vi "CMI ADS127L21 - Get Error.vi"(8 "error in (no error)":errorcluster, 10 "Read All? (true)":bool=TRUE, 11 "VISA in":refnum<visa-resource-name>) -> (0 "error out":errorcluster, 3 "VISA out":refnum<visa-resource-name>)   [LabVIEW 2020]
doc: "Open digitizer."
uses:
  <vilib>/Instr/_visa.llb/VISA Flush IO Buffer Mask.ctl
  <vilib>/Utility/error.llb/Error Cluster From Error Code.vi
  <vilib>/ErrorRing/Error Ring.xnode
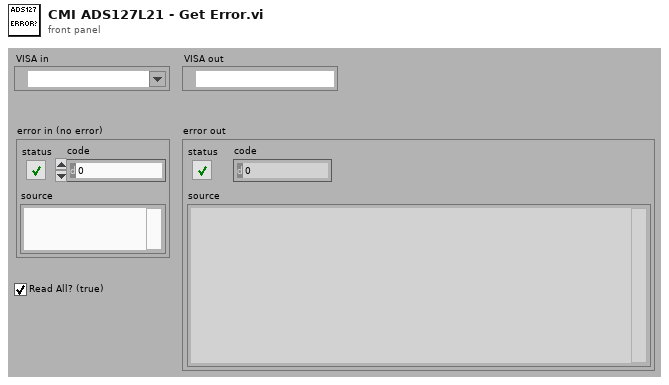
[diagram p1: front panel]
types:
  T1 = typedef "VISA Flush IO Buffer Mask.ctl" = u16
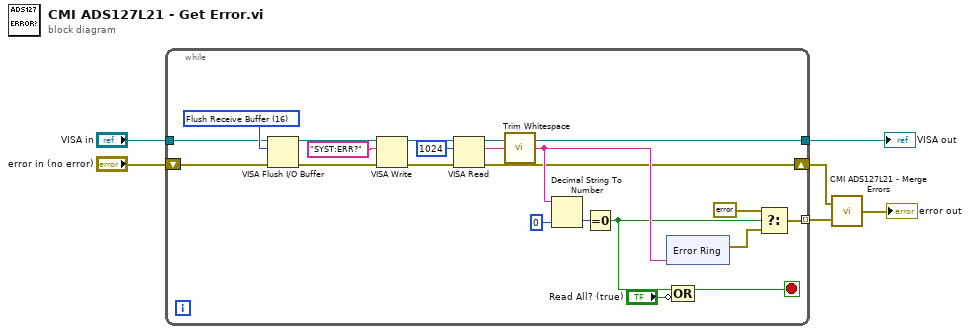
[diagram p0: block diagram]
diagram:
  n1 = while {
    tunnel: "VISA in" -> [w18]
    tunnel: [w11] -> w4 mode=indexing
    shift-right: [w12] -> w2
    shift-left: "error in (no error)" -> [w19]
    tunnel: [w10] -> w1
    stop <- w8 stop-if-true
    w27 = T1 16 items=["Flush Receive Buffer"=16, "Write Transmit Buffer to Device"=32, "Flush Receive Buffer (No I/O)"=64, "Flush Transmit Buffer"=128] ("Mask")
    n2 = VISA Flush I/O Buffer(VISA resource name=w18, mask (16)=w27, error in (no error)=w19) -> (VISA resource name out=w25:refnum<visa-resource-name>, error out=w26:errorcluster)
    n3 = VISA Write(VISA resource name=w25, write buffer="SYST:ERR?", error in (no error)=w26) -> (VISA resource name out=w22:refnum<visa-resource-name>, error out=w23:errorcluster)  [unwired: 1 out]
    n4 = VISA Read(VISA resource name=w22, byte count=u32 1024, error in (no error)=w23) -> (VISA resource name out=w10:refnum<visa-resource-name>, read buffer=w20:string, error out=w12:errorcluster)  [unwired: 1 out]
    n5 = call <vilib>:"Trim Whitespace.vi"("string"=w20) -> ("trimmed string"=w17:string)  [unwired: 1 in]
    n6 = Decimal String To Number(string=w17, default (0L)=0 ("default (0 I32)")) -> (number=w15:i32)  [unwired: 1 in, 1 out]
    n7 = Equal To 0?(x=w15) -> (x = 0?=w9:bool)
    n8 = xnode "Error Ring"("parameter 0"=w17) -> ("error out"=w13:errorcluster)
    n9 = Compound Arithmetic op=OR(w9, invert "Read All? (true)") -> (w8:bool)
    n10 = Select(t=errorcluster {"status"=FALSE, "code"=0, "source"=""} ("f"), s=w9, f=w13) -> (s? t:f=w11:errorcluster)
  }
  "VISA out" <- w1
  n11 = call "CMI ADS127L21 - Merge Errors.vi"("errors in"=w4, "error in (no error)"=w2) -> ("error out"=→"error out":errorcluster)
